vi "Close.vi"(8 "error in (no error)":errorcluster, 11 "Pickering in":refnum<class "Pickering.lvclass">) -> (0 "error out":errorcluster, 3 "Pickering out":refnum<class "Pickering.lvclass">)   [LabVIEW 2019, in "Pickering.lvclass"]
uses:
  Pickering.lvclass
  InstrumentSetup.vi
  InstrControl.lvclass
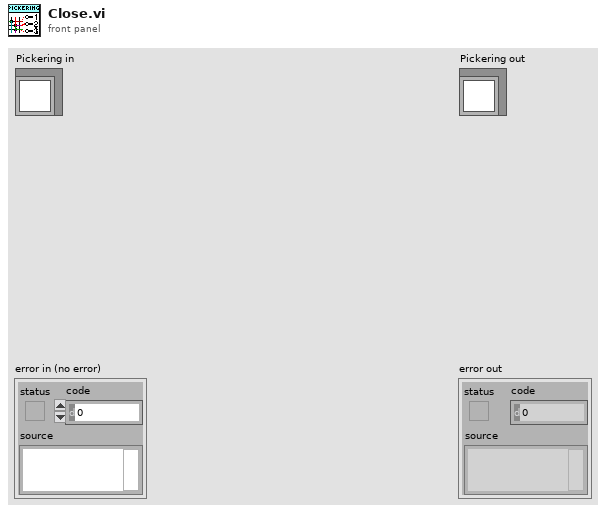
[diagram p1: front panel]
types:
  T1 = cluster{"KE 2410":cluster{"Instrument name":string, "address":refnum<visa-resource-name>, "Instrument type":u16}, "KE 6517":cluster{"Instrument name":string, "address":refnum<visa-resource-name>, "Instrument type":u16}, "KE 487":cluster{"Instrument name":string, "address":refnum<visa-resource-name>, "Instrument type":u16}, "KE 236":cluster{"Instrument name":string, "address":refnum<visa-resource-name>, "Instrument type":u16}, "WK 6440B":cluster{"Instrument name":string, "address":refnum<visa-resource-name>, "Instrument type":u16}, "WK 6425":cluster{"Instrument name":string, "address":refnum<visa-resource-name>, "Instrument type":u16}, "Pickering Matrix":cluster{"Instrument name":string, "address":refnum<visa-resource-name>, "Instrument type":u16}, "KE 2000":cluster{"Instrument name":string, "address":refnum<visa-resource-name>, "Instrument type":u16}, "KE3706A Switching":cluster{"Instrument name":string, "address":refnum<visa-resource-name>, "Instrument type":u16}, "KE 2657A":cluster{"Instrument name":string, "address":refnum<visa-resource-name>, "Instrument type":u16}, "R_METAL KE2410":cluster{"Instrument name":string, "address":refnum<visa-resource-name>, "Instrument type":u16}, "HP34401A":cluster{"Instrument name":string, "address":refnum<visa-resource-name>, "Instrument type":u16}}
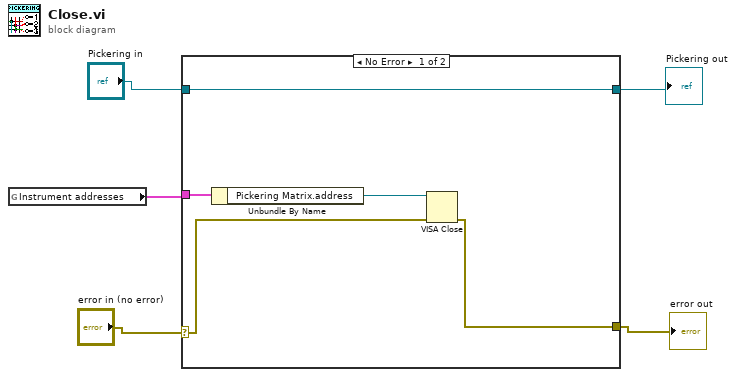
[diagram p0: block diagram]
diagram:
  n1 = global read "InstrumentSetup.vi" "Instrument addresses"() -> (w1:T1)
  n2 = case shown="No Error" "error in (no error)" {
    selector: "error in (no error)" -> [w8 w12]
    tunnel: w1 -> [w10 _]
    tunnel: [w7 w12] -> w4
    tunnel: [w6 w11] -> w2
    tunnel: "Pickering in" -> [w6 w11]
    frame No Error {
      n3 = Unbundle By Name(w10) -> ("Pickering Matrix.address"=w9:refnum<visa-resource-name>)
      n4 = VISA Close(VISA resource name=w9, error in (no error)=w8) -> (error out=w7:errorcluster)
    }
    frame Error {
    }
  }
  "error out" <- w4
  "Pickering out" <- w2
